vi "Sel UnSel a Item.vi"(8 "error in (no error)":errorcluster, 10 "Coords":cluster{"Horizontal":i32, "Vertical":i32}, 11 "Methods ListCtrl":refnum<vi>) -> (0 "error out":errorcluster, 3 "Methods ListCtrl 2":refnum<vi>)   [LabVIEW 2017, in "WebServiceImporter.lvlib" / "Main Panel.lvlib" / "Select Methods.lvlib"]
uses:
  <vilib>/Platform/WebService/Main Panel/Pages/Select Methods/Select Methods.lvlib
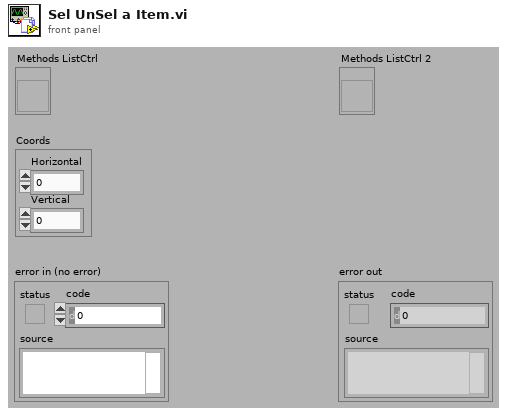
[diagram p1: front panel]
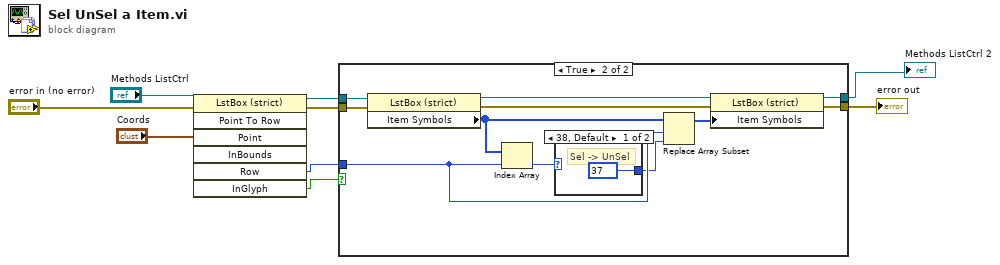
[diagram p0: block diagram]
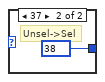
[diagram p3: hidden frame]
diagram:
  n1 = invoke class="LstBox (strict)" method="Point To Row"(reference="Methods ListCtrl", error in="error in (no error)", "Point"="Coords") -> (reference out=w6:refnum<vi>, error out=w5:errorcluster, "Row"=w4:i32, "InGlyph"=w7:bool)  [unwired: 4 in, 3 out]
  n2 = case shown="True" w7 {
    tunnel: w6 -> [w10 w22]
    tunnel: w5 -> [w11 w21]
    tunnel: w4 -> [_ w18]
    tunnel: [w11 w13] -> w3
    tunnel: [w10 w12] -> w1
    frame False {
    }
    frame True {
      n3 = property class="LstBox (strict)"(reference=w22, error in=w21) -> (reference out=w16:refnum<vi>, error out=w15:errorcluster, "Item Symbols"=w20:i32[])
      n4 = Index Array(array=w20, index=w18) -> (element=w19:i32)
      n5 = case shown="38, Default" w19 {
        tunnel: [37 38] -> w17
        frame 38, Default {
          # "Sel -> UnSel"
        }
        frame 37 {
          # "Unsel->Sel"
        }
      }
      n6 = Replace Array Subset(array=w20, new element=w17, index=w18) -> (w14:i32[])
      n7 = property class="LstBox (strict)"(reference=w16, error in=w15, "Item Symbols"=w14) -> (reference out=w12:refnum<vi>, error out=w13:errorcluster)
    }
  }
  "error out" <- w3
  "Methods ListCtrl 2" <- w1
